vi "tcpServerStateMachine.vi"(8 "error in (no error)":errorcluster, 9 "notifierTcpConn":refnum<notifier>, 10 "queueTcpServer":refnum<queue>, 11 "TcpServerCmd in":refnum<class "TcpServerCmd.lvclass">) -> (0 "error out":errorcluster, 3 "TcpServerCmd out":refnum<class "TcpServerCmd.lvclass">)   [LabVIEW 2018, in "TcpServerCmd.lvclass"]
doc: "TCP Server State Machine. The execution is set as Preallocated Reentrant Execution Function. This is for the two runServer.vi child functions to have two different clones.\n\nStates:\n\n1.- Create Listener.\n2.- Wait on Listener.\n3.- Read TCP Packet.\n4.- Close Connection.\n5.- Stop Server."
uses:
  TcpServerCmd.lvclass
  home/pcortes/github/ts_labview_tcp_json/src/TcpServerBase/TcpServerBase.lvclass
  TcpServerBase/TcpServerBase.lvclass/TcpServerBase.ctl
  TcpServerBase/typedef/tcpConnectionTypeDef.ctl
  TcpServerCmd.lvclass/TcpServerCmd.ctl
  TcpServerBase/TcpServerBase.lvclass
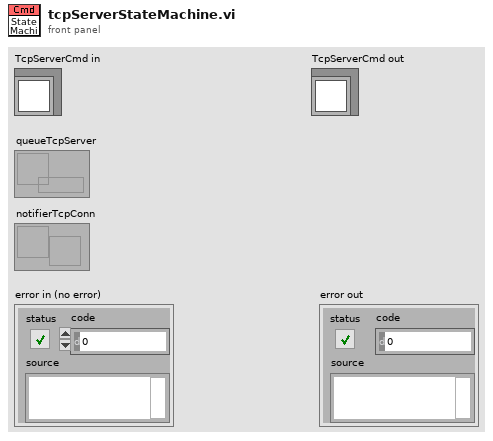
[diagram p1: front panel]
types:
  T1 = typedef "TcpServerBase.lvclass/tcpConnectionTypeDef.ctl" = cluster{"connection ID":refnum<k5>, "firstConnection":bool}
  T2 = enum16{"Standard", "Buffered", "CRLF", "Immediate"}
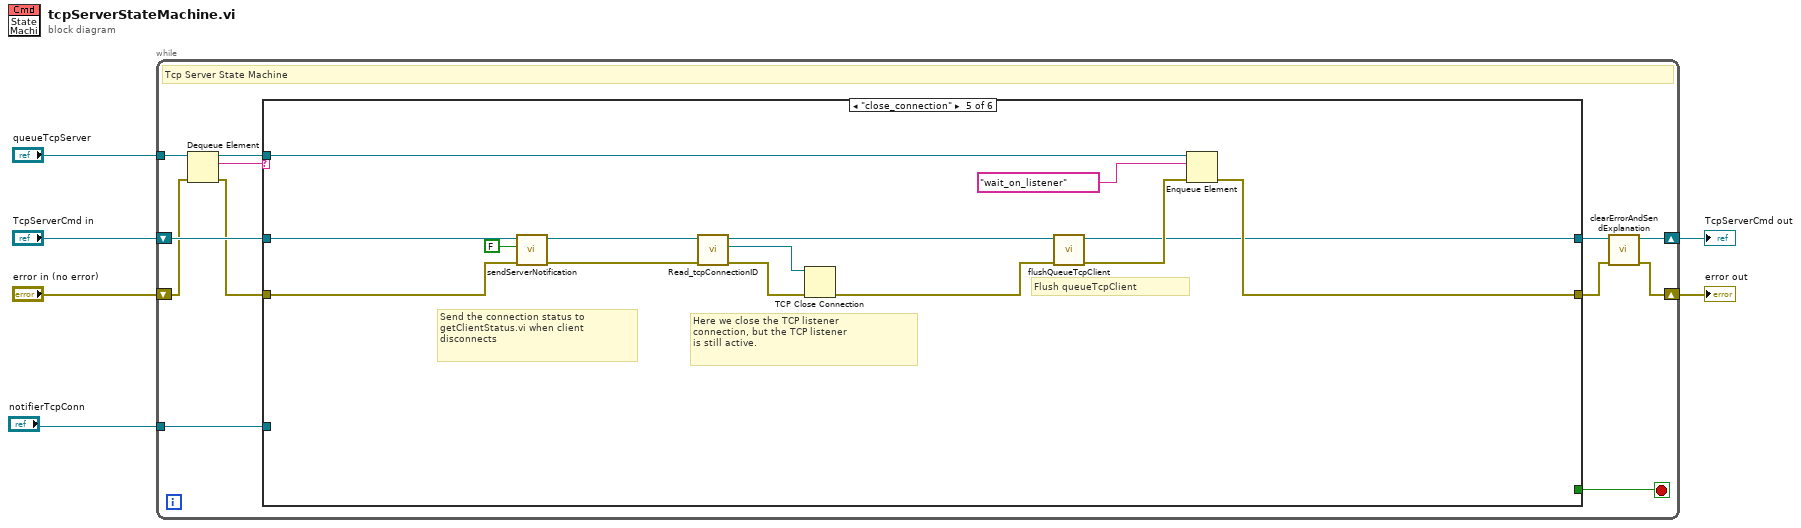
[diagram p0: block diagram]
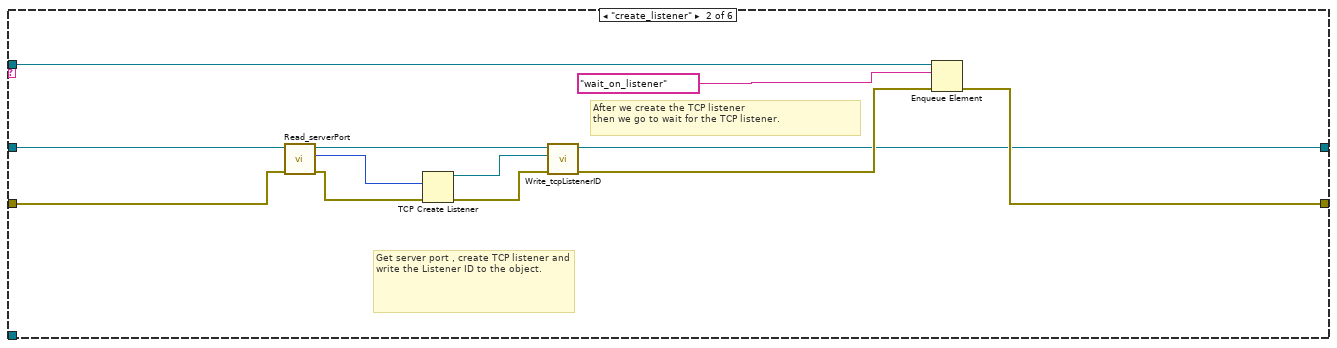
[diagram p3: hidden frame]
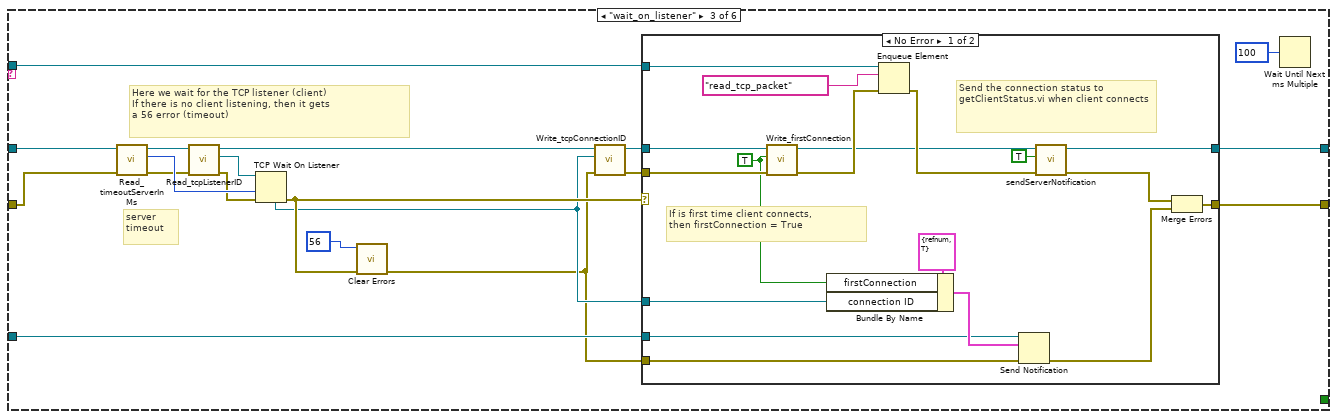
[diagram p4: hidden frame]
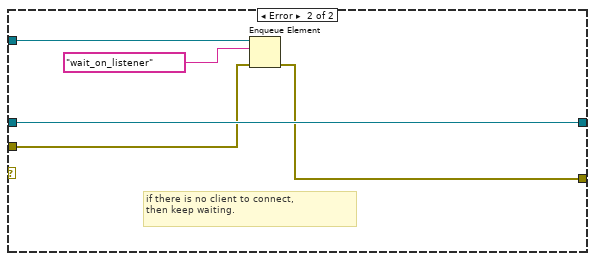
[diagram p5: hidden frame]
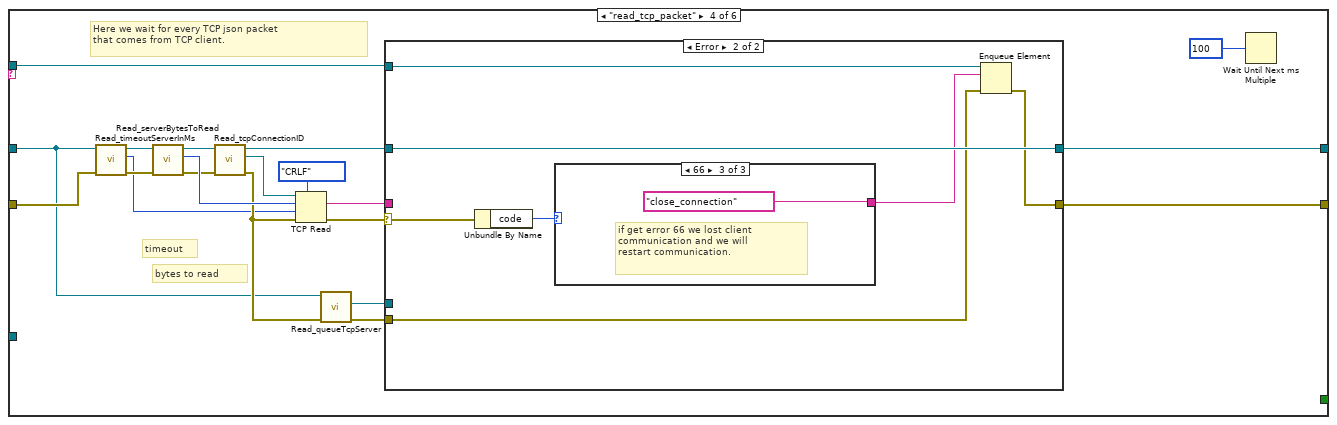
[diagram p6: hidden frame]
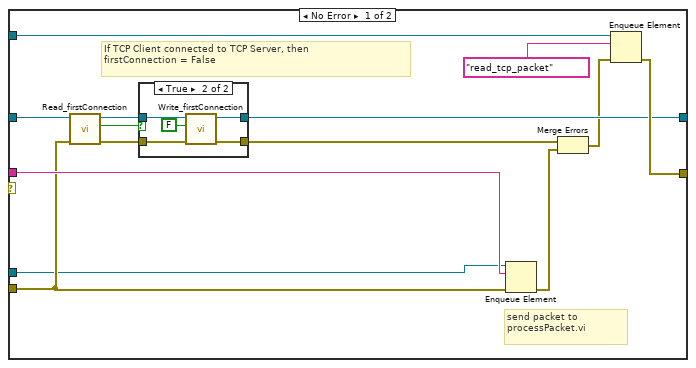
[diagram p7: hidden frame]
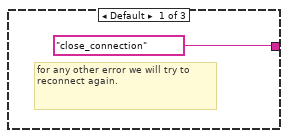
[diagram p9: hidden frame]
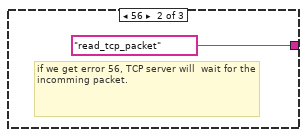
[diagram p10: hidden frame]
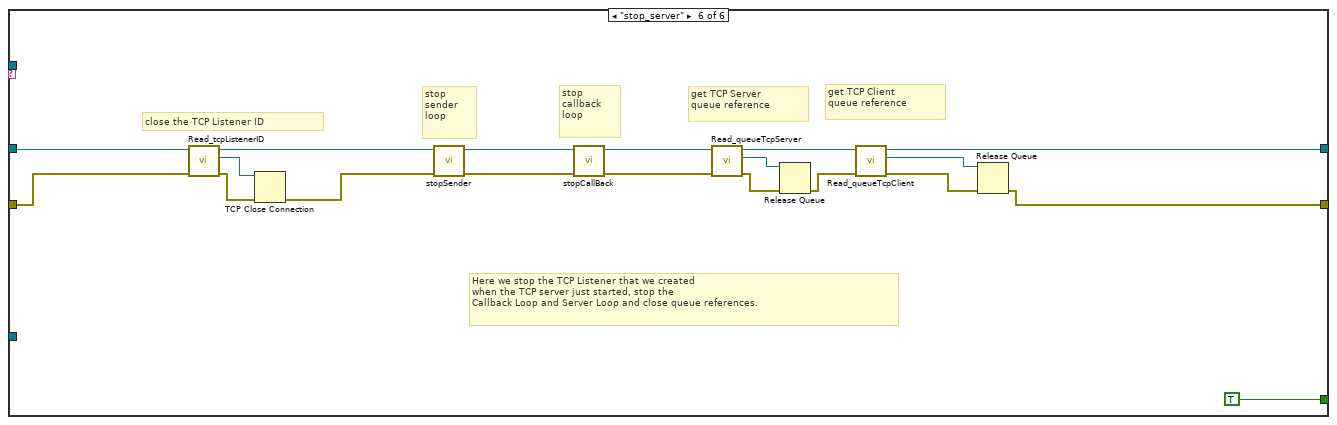
[diagram p11: hidden frame]
diagram:
  n1 = while {
    tunnel: "queueTcpServer" -> [w18]
    shift-right: [w7] -> w3
    shift-left: "TcpServerCmd in" -> [w17]
    shift-right: [w9] -> w6
    shift-left: "error in (no error)" -> [w12]
    tunnel: "notifierTcpConn" -> [w10]
    stop <- w14 stop-if-true
    # "Tcp Server State Machine"
    n2 = Dequeue Element(queue=w18, error in (no error)=w12) -> (queue out=w16:refnum<queue>, element=w15:string, error out=w11:errorcluster)  [unwired: 1 in, 1 out]
    n3 = case shown="\"close_connection\"" w15 {
      tunnel: w17 -> [w20 w30 w48 w76 w132 w157]
      tunnel: [w20 w21 w47 w88 w126 w152] -> w8
      tunnel: w16 -> [_ w26 w46 w81 w139 _]
      tunnel: [_ _ _ _ _ TRUE] -> w14
      tunnel: w11 -> [w19 w24 w44 w86 w136 w151]
      tunnel: [w19 w22 w38 w80 w134 w144] -> w13
      tunnel: w10 -> [_ _ w35 _ _ _]
      frame Default {
        # "Do notihig for now."
      }
      frame "create_listener" {
        # "After we create the TCP listener\nthen we go to wait for the TCP listener."
        # "Get server port , create TCP listener and write the Listener ID to the object."
        n4 = call "Read_serverPort.vi"("error in (no error)"=w24, "TcpServerBase in"=w30) -> ("error out"=w31:errorcluster, "serverPort"=w32:u16, "TcpServerBase out"=w29:refnum<class "TcpServerCmd.lvclass">)  [unwired: 7 in]
        n5 = TCP Create Listener(8:w31, 10:w32) -> (0:w27:errorcluster, 3:w28:refnum<k5>)  [unwired: 3 in, 1 out]
        n6 = call "Write_tcpListenerID.vi"("error in (no error)"=w27, "tcpListenerID"=w28, "TcpServerBase in"=w29) -> ("error out"=w23:errorcluster, "TcpServerBase out"=w21:refnum<class "TcpServerCmd.lvclass">)  [unwired: 7 in]
        n7 = Enqueue Element(queue=w26, element="wait_on_listener", error in (no error)=w23) -> (error out=w22:errorcluster)  [unwired: 1 in, 2 out]
      }
      frame "wait_on_listener" {
        # "Here we wait for the TCP listener (client)\nIf there is no client listening, then it gets\na 56 error (timeout)"
        # "server\ntimeout"
        n8 = call "Read_timeoutServerInMs.vi"("error in (no error)"=w44, "TcpServerBase in"=w48) -> ("error out"=w43:errorcluster, "timeoutServerInMs"=w49:i32, "TcpServerBase out"=w50:refnum<class "TcpServerCmd.lvclass">)  [unwired: 7 in]
        n9 = call "Read_tcpListenerID.vi"("error in (no error)"=w43, "TcpServerBase in"=w50) -> ("error out"=w42:errorcluster, "tcpListenerID"=w51:refnum<k5>, "TcpServerBase out"=w36:refnum<class "TcpServerCmd.lvclass">)  [unwired: 7 in]
        n10 = TCP Wait On Listener(8:w42, 9:w49, 11:w51) -> (0:w40:errorcluster, 4:w34:refnum<k5>)  [unwired: 1 in, 3 out]
        n11 = call <vilib>:"Clear Errors.vi"("error in (no error)"=w40, "specific error code to clear (0: all)"=56) -> ("error out"=w33:errorcluster)  [unwired: 4 in, 1 out]
        n12 = call "Write_tcpConnectionID.vi"("error in (no error)"=w33, "tcpConnectionID"=w34, "TcpServerBase in"=w36) -> ("error out"=w39:errorcluster, "TcpServerBase out"=w45:refnum<class "TcpServerCmd.lvclass">)  [unwired: 7 in]
        n13 = case shown="No Error" w40 {
          tunnel: w45 -> [w64 w74]
          tunnel: [w53 w74] -> w47
          tunnel: w46 -> [w68 w73]
          tunnel: w39 -> [w67 w71]
          tunnel: [w57 w70] -> w38
          tunnel: w35 -> [w61 _]
          tunnel: w34 -> [w59 _]
          tunnel: w33 -> [w58 _]
          frame No Error {
            w60 = TRUE ("firstConnection")
            # "Send the connection status to getClientStatus.vi when client connects"
            # "If is first time client connects,\nthen firstConnection = True"
            n14 = call "Write_firstConnection.vi"("error in (no error)"=w67, "firstConnection"=w60, "TcpServerCmd in"=w64) -> ("error out"=w66:errorcluster, "TcpServerCmd out"=w54:refnum<class "TcpServerCmd.lvclass">)  [unwired: 7 in]
            n15 = Bundle By Name(cluster=T1 {"connection ID"=refnum, "firstConnection"=TRUE} ("TcpConnectionCluster"), "firstConnection"=w60, "connection ID"=w59) -> (w63:T1)
            n16 = Enqueue Element(queue=w68, element="read_tcp_packet", error in (no error)=w66) -> (error out=w65:errorcluster)  [unwired: 1 in, 2 out]
            n17 = Send Notification(notification=w63, notifier=w61, error in (no error)=w58) -> (error out=w56:errorcluster)  [unwired: 1 out]
            n18 = call "sendServerNotification.vi"("error in (no error)"=w65, "connectionStatus"=TRUE ("serverStatus"), "TcpServerBase in"=w54) -> ("error out"=w55:errorcluster, "TcpServerBase out"=w53:refnum<class "TcpServerCmd.lvclass">)  [unwired: 7 in]
            n19 = Merge Errors(w55, w56) -> (w57:errorcluster)
          }
          frame Error {
            # "if there is no client to connect, \nthen keep waiting."
            n20 = Enqueue Element(queue=w73, element="wait_on_listener", error in (no error)=w71) -> (error out=w70:errorcluster)  [unwired: 1 in, 2 out]
          }
        }
        n21 = Wait Until Next ms Multiple(millisecond multiple=u32 100) -> ()  [unwired: 1 out]
      }
      frame "read_tcp_packet" {
        # "timeout"
        # "Here we wait for every TCP json packet\nthat comes from TCP client."
        # "bytes to read"
        n22 = call "Read_timeoutServerInMs.vi"("error in (no error)"=w86, "TcpServerBase in"=w76) -> ("error out"=w78:errorcluster, "timeoutServerInMs"=w75:i32, "TcpServerBase out"=w77:refnum<class "TcpServerCmd.lvclass">)  [unwired: 7 in]
        n23 = call "Read_serverBytesToRead.vi"("error in (no error)"=w78, "TcpServerBase in"=w77) -> ("error out"=w87:errorcluster, "serverBytesToRead"=w91:i32, "TcpServerBase out"=w90:refnum<class "TcpServerCmd.lvclass">)  [unwired: 7 in]
        n24 = call "Read_tcpConnectionID.vi"("error in (no error)"=w87, "TcpServerBase in"=w90) -> ("error out"=w83:errorcluster, "tcpConnectionID"=w79:refnum<k5>, "TcpServerBase out"=w89:refnum<class "TcpServerCmd.lvclass">)  [unwired: 7 in]
        n25 = TCP Read(connection ID=w79, bytes to read=w91, error in (no error)=w83, 7:T2."CRLF" ("mode (standard)"), 9:w75) -> (data out=w94:string, error out=w92:errorcluster)  [unwired: 1 out]
        n26 = call "Read_queueTcpServer.vi"("error in (no error)"=w83, "TcpServerBase in"=w76) -> ("error out"=w82:errorcluster, "queueTcpServer"=w85:refnum<queue>)  [unwired: 7 in, 1 out]
        n27 = case shown="Error" w92 {
          selector: w92 -> [_ w122]
          tunnel: w94 -> [w108 _]
          tunnel: w85 -> [w95 _]
          tunnel: w89 -> [w101 w120]
          tunnel: [w102 w120] -> w88
          tunnel: w82 -> [w96 w117]
          tunnel: w81 -> [w107 w119]
          tunnel: [w105 w116] -> w80
          frame No Error {
            # "If TCP Client connected to TCP Server, then\nfirstConnection = False"
            # "send packet to\nprocessPacket.vi"
            n28 = call "Read_firstConnection.vi"("error in (no error)"=w96, "TcpServerCmd in"=w101) -> ("error out"=w104:errorcluster, "firstConnection"=w100:bool, "TcpServerCmd out"=w103:refnum<class "TcpServerCmd.lvclass">)  [unwired: 7 in]
            n29 = case shown="True" w100 {
              tunnel: w104 -> [w109 w115]
              tunnel: [w109 w114] -> w99
              tunnel: w103 -> [w110 w113]
              tunnel: [w110 w112] -> w102
              frame False {
              }
              frame True {
                n30 = call "Write_firstConnection.vi"("error in (no error)"=w115, "firstConnection"=FALSE, "TcpServerCmd in"=w113) -> ("error out"=w114:errorcluster, "TcpServerCmd out"=w112:refnum<class "TcpServerCmd.lvclass">)  [unwired: 7 in]
              }
            }
            n31 = Enqueue Element(queue=w95, element=w108, error in (no error)=w96) -> (error out=w98:errorcluster)  [unwired: 1 in, 2 out]
            n32 = Merge Errors(w99, w98) -> (w97:errorcluster)
            n33 = Enqueue Element(queue=w107, element="read_tcp_packet", error in (no error)=w97) -> (error out=w105:errorcluster)  [unwired: 1 in, 2 out]
          }
          frame Error {
            n34 = Unbundle By Name(w122) -> ("code"=w121:i32)
            n35 = case shown="66" w121 {
              tunnel: ["close_connection" "read_tcp_packet" "close_connection"] -> w118
              frame Default {
                # "for any other error we will try to reconnect again."
              }
              frame 56 {
                # "if we get error 56, TCP server will  wait for the incomming packet."
              }
              frame 66 {
                # "if get error 66 we lost client \ncommunication and we will\nrestart communication."
              }
            }
            n36 = Enqueue Element(queue=w119, element=w118, error in (no error)=w117) -> (error out=w116:errorcluster)  [unwired: 1 in, 2 out]
          }
        }
        n37 = Wait Until Next ms Multiple(millisecond multiple=u32 100) -> ()  [unwired: 1 out]
      }
      frame "close_connection" {
        # "Flush queueTcpClient"
        # "Send the connection status to getClientStatus.vi when client disconnects"
        # "Here we close the TCP listener\nconnection, but the TCP listener\nis still active."
        n38 = call "sendServerNotification.vi"("error in (no error)"=w136, "connectionStatus"=FALSE ("serverStatus"), "TcpServerBase in"=w132) -> ("error out"=w133:errorcluster, "TcpServerBase out"=w131:refnum<class "TcpServerCmd.lvclass">)  [unwired: 7 in]
        n39 = call "Read_tcpConnectionID.vi"("error in (no error)"=w133, "TcpServerBase in"=w131) -> ("error out"=w135:errorcluster, "tcpConnectionID"=w137:refnum<k5>, "TcpServerBase out"=w129:refnum<class "TcpServerCmd.lvclass">)  [unwired: 7 in]
        n40 = TCP Close Connection(connection ID=w137, error in (no error)=w135) -> (error out=w128:errorcluster)  [unwired: 1 in, 1 out]
        n41 = call "flushQueueTcpClient.vi"("error in (no error)"=w128, "TcpServerBase in"=w129) -> ("error out"=w127:errorcluster, "TcpServerBase out"=w126:refnum<class "TcpServerCmd.lvclass">)  [unwired: 8 in]
        n42 = Enqueue Element(queue=w139, element="wait_on_listener", error in (no error)=w127) -> (error out=w134:errorcluster)  [unwired: 1 in, 2 out]
      }
      frame "stop_server" {
        # "stop\ncallback\nloop"
        # "stop\nsender\nloop"
        # "Here we stop the TCP Listener that we created\nwhen the TCP server just started, stop the \nCallback Loop and Server Loop and close queue references."
        # "close the TCP Listener ID"
        # "get TCP Client \nqueue reference"
        # "get TCP Server \nqueue reference"
        n43 = call "Read_tcpListenerID.vi"("error in (no error)"=w151, "TcpServerBase in"=w157) -> ("error out"=w150:errorcluster, "tcpListenerID"=w158:refnum<k5>, "TcpServerBase out"=w143:refnum<class "TcpServerCmd.lvclass">)  [unwired: 7 in]
        n44 = TCP Close Connection(connection ID=w158, error in (no error)=w150) -> (error out=w149:errorcluster)  [unwired: 1 in, 1 out]
        n45 = call "stopSender.vi"("error in (no error)"=w149, "TcpServerBase in"=w143) -> ("error out"=w140:errorcluster, "TcpServerBase out"=w141:refnum<class "TcpServerCmd.lvclass">)  [unwired: 8 in]
        n46 = call "stopCallBack.vi"("error in (no error)"=w140, "TcpServerBase in"=w141) -> ("error out"=w148:errorcluster, "TcpServerBase out"=w142:refnum<class "TcpServerCmd.lvclass">)  [unwired: 8 in]
        n47 = call "Read_queueTcpServer.vi"("error in (no error)"=w148, "TcpServerBase in"=w142) -> ("error out"=w147:errorcluster, "queueTcpServer"=w155:refnum<queue>, "TcpServerBase out"=w154:refnum<class "TcpServerCmd.lvclass">)  [unwired: 7 in]
        n48 = Release Queue(queue=w155, error in (no error)=w147) -> (error out=w146:errorcluster)  [unwired: 1 in, 2 out]
        n49 = call "Read_queueTcpClient.vi"("error in (no error)"=w146, "TcpServerBase in"=w154) -> ("error out"=w145:errorcluster, "queueTcpClient"=w153:refnum<queue>, "TcpServerBase out"=w152:refnum<class "TcpServerCmd.lvclass">)  [unwired: 7 in]
        n50 = Release Queue(queue=w153, error in (no error)=w145) -> (error out=w144:errorcluster)  [unwired: 1 in, 2 out]
      }
    }
    n51 = call "clearErrorAndSendExplanation.vi"("error in (no error)"=w13, "TcpServerBase in"=w8) -> ("error out"=w9:errorcluster, "TcpServerBase out"=w7:refnum<class "TcpServerCmd.lvclass">)  [unwired: 8 in]
  }
  "error out" <- w6
  "TcpServerCmd out" <- w3
